vi "Configure.vi"(8 "error in (no error)":errorcluster, 11 "Cascade in":refnum<class "Cascade.lvclass">) -> (0 "error out":errorcluster, 2 "cancelled?":bool, 3 "Cascade out":refnum<class "Cascade.lvclass">)   [LabVIEW 2012, in "Cascade.lvclass"]
doc: "The configure method configures the details for the RabbitMQ connection, the observers and the mapping script.\n\nIn the derived class, make a call to the parent for setting these parameters."
uses:
  Cascade.lvclass
  timing mode.ctl
  Trigger edge.ctl
  acquire flag.ctl
  gain mode.ctl
  dependencies/ImageReg/Edge and object parameters.ctl
  dependencies/ImageReg/Registration method.ctl
  dependencies/ImageReg/BinarizationParameters.ctl
  dependencies/ImageReg/Gaussian blur parameters.ctl
  <vilib>/Utility/miscctls.llb/LVPointTypeDef.ctl
  Cascade.lvclass/Cascade.ctl
  <vilib>/Distrio/Murmex/Murmex/Murmex.lvclass
panel:
  in  "Tab Control":T1(tab)
  in  "Accumulations":u32
  in  "Number of frames":u32
  in  "Temperature":dbl=-70.0
  in  "Gain mode":T2 items=["Safe mode"=1, "Gate mode"=2, "Shutter mode"=3]
  in  "Acquire flag":T3 items=["Sync Focus mode"=1, "Sync N Frame mode"=2, "Async mode"=3, "Sequence moce"=4]
  in  "Timing mode":T4 items=["Free run"=1, "External trigger"=2, "Strobe mode  (ext trigger)"=3, "Bulb mode (ext trigger)"=4, "Variable mode (ext trigger)"=5, "Flash mdoe (ext trigger)"=6]
  in  "Trigger Edge":T5 items=["Leading edge"=1, "Falling edge"=2]
  in  "LUT":path
  in  "Background image":path
  in  "Gaussian blur parameters":T6={"large sigma"=20.0, "small sigma"=4.0, "equalize?"=FALSE}
  in  "Binarization parameters":T7={"threshold percentage"=95.0, "equalize?"=FALSE, "Method (clustering)"=0} {"Method (clustering)" items=["clustering", "entropy", "metric", "moments", "inter-class variance"]}
  in  "min physical displacement":dbl[unit]
  in  "max physical displacement":dbl[unit]
  in  "saturation limit":dbl
  in  "Registration method":T8
  in  "min y pixel displ.":dbl
  in  "max y pixel displ.":dbl
  in  "max pixel discrepancy":dbl
  in  "min x pixel displ.":dbl
  in  "max x pixel displ.":dbl
  in  "micron equivalent of pixel":dbl[unit]
  in  "brightness threshold":sgl
  in  "stage component":string
  in  "Edge and object Parameters":T9={"Canny Edge Parameters"={"Sigma"=1.0, "HThresh"=0.7, "LThres"=0.2, "WindowSize"=9}, "Smoothing parameters"={"X Size"=3, "Y Size"=3, "% Tolerance"=40}, "Dilation iteration"=1, "Object recognition parameters"={"Objects"=0, "Threshold"=128, "Reject Border"=FALSE, "Fill Holes"=FALSE, "Min Object Size"=FALSE, "Min Size"=3, "Max Object Size"=FALSE, "Max Size"=100, "Show Search Area"=FALSE, "Show Center"=TRUE, "Show Bounding Box"=TRUE}} {"Object recognition parameters"."Objects" items=["Bright Objects", "Dark Objects"]; "Object recognition parameters"."Threshold" min=1 max=999999999 step=1; "Object recognition parameters"."Max Size" min=1 max=999999999 step=1; "Object recognition parameters"."Min Size" min=1 max=999999999 step=1; "Canny Edge Parameters"."LThres" min=0 max=1 format="%.2f"; "Canny Edge Parameters"."HThresh" min=0 max=1 format="%.2f"; "Canny Edge Parameters"."Sigma" min=0 max=1 format="%.2f"}
  in  "button:call parent":bool
  in  "button:ok":bool
  in  "button:cancel":bool
  # "RabbitMQ parameters"
  # "Window position"
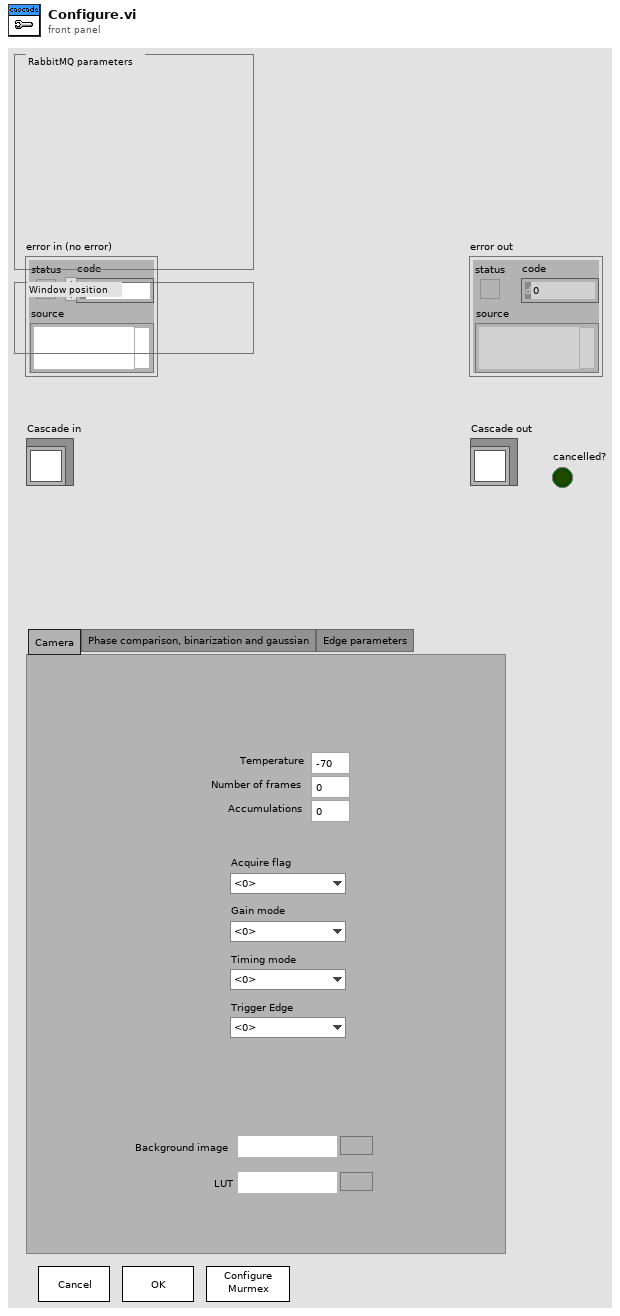
[diagram p1: front panel]
types:
  T1 = enum32{"Camera", "Phase comparison, binarization and gaussian", "Edge parameters"}
  T2 = typedef "Cascade.lvclass/gain mode.ctl" = u32
  T3 = typedef "Cascade.lvclass/acquire flag.ctl" = u32
  T4 = typedef "Cascade.lvclass/timing mode.ctl" = u32
  T5 = typedef "Cascade.lvclass/Trigger edge.ctl" = u32
  T6 = typedef "Gaussian blur parameters.ctl" = cluster{"large sigma":sgl, "small sigma":sgl, "equalize?":bool}
  T7 = typedef "BinarizationParameters.ctl" = cluster{"threshold percentage":dbl, "equalize?":bool, "Method (clustering)":i32}
  T8 = typedef "Registration method.ctl" = enum16{"Binarization", "Difference of Gaussians", "Edges Detection", "Gaussians and Binarization", "Edges and Gaussians", "Edges and Binarization", "All"}
  T9 = typedef "Edge and object parameters.ctl" = cluster{"Canny Edge Parameters":cluster{"Sigma":sgl, "HThresh":sgl, "LThres":sgl, "WindowSize":i32}, "Smoothing parameters":cluster{"X Size":i32, "Y Size":i32, "% Tolerance":i32}, "Dilation iteration":i32, "Object recognition parameters":cluster{"Objects":u16, "Threshold":i32, "Reject Border":bool, "Fill Holes":bool, "Min Object Size":bool, "Min Size":i32, "Max Object Size":bool, "Max Size":i32, "Show Search Area":bool, "Show Center":bool, "Show Bounding Box":bool}}
  T10 = typedef "LVPointTypeDef.ctl" = cluster{"Horizontal":i16, "Vertical":i16}
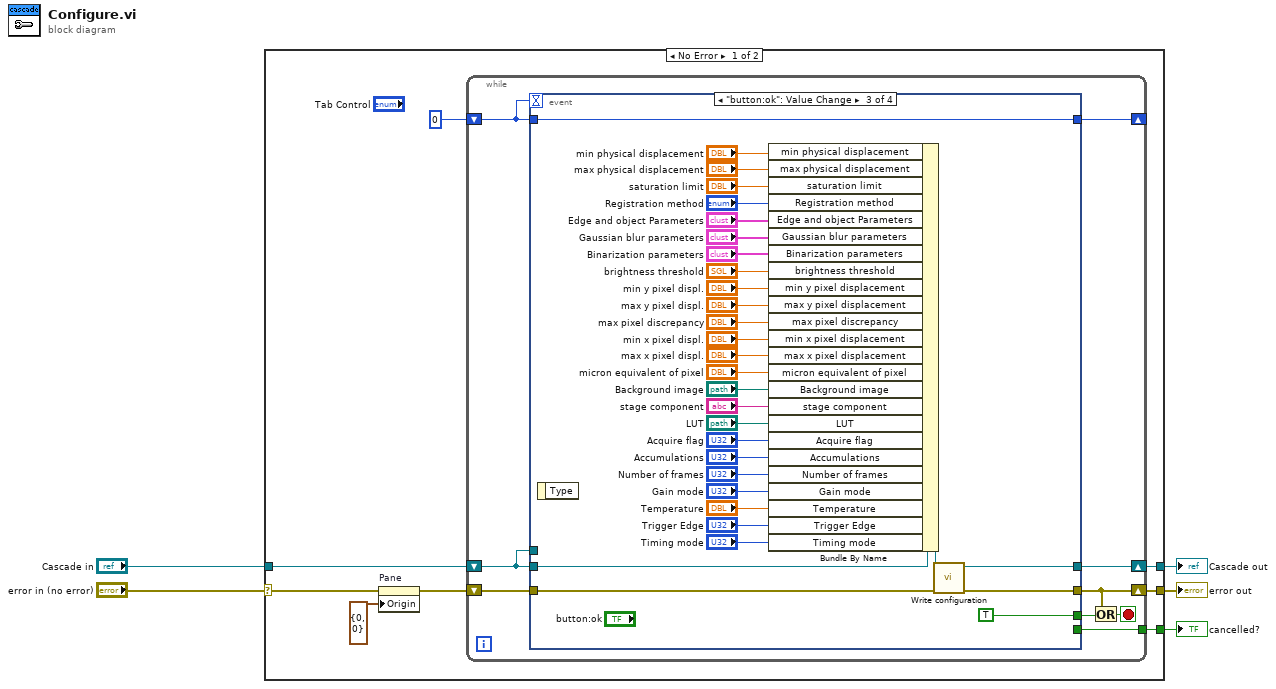
[diagram p0: block diagram]
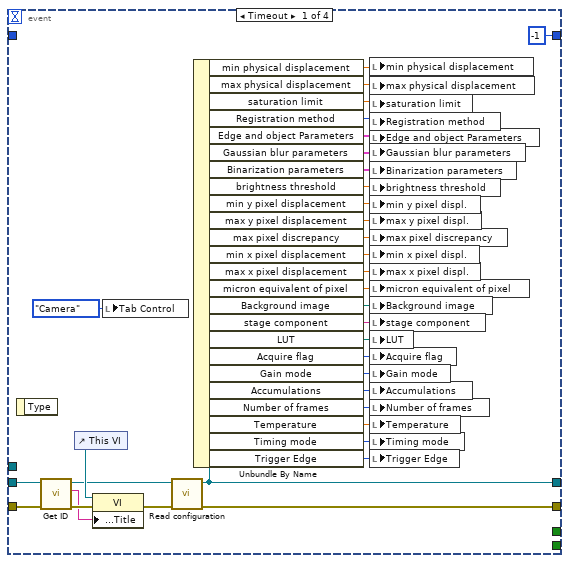
[diagram p2: hidden frame]
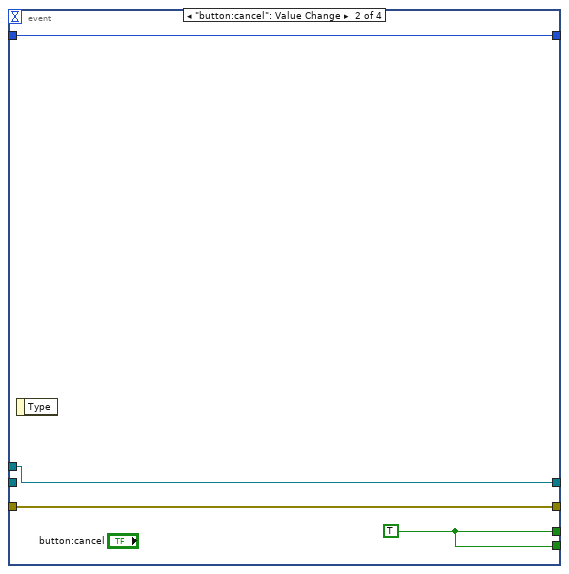
[diagram p3: hidden frame]
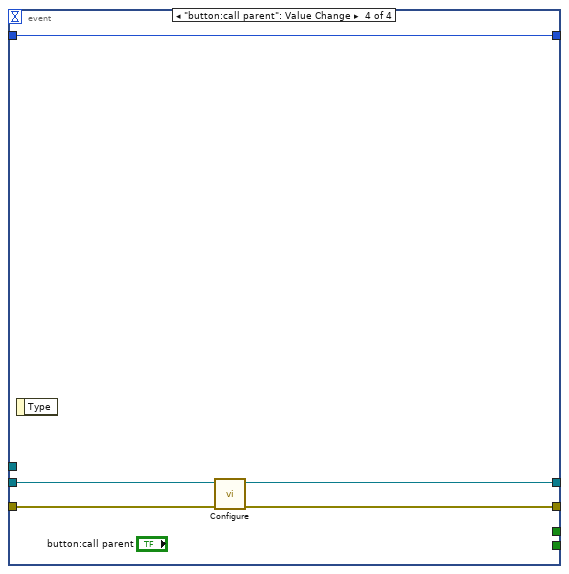
[diagram p4: hidden frame]
diagram:
  n1 = case shown="No Error" "error in (no error)" {
    selector: "error in (no error)" -> [w12 w98]
    tunnel: "Cascade in" -> [w9 w99]
    tunnel: [w10 w98] -> w3
    tunnel: [w7 w99] -> w2
    tunnel: [w6 _] -> w1
    frame No Error {
      n2 = property on="Pane" class="Pane"(error in=w12, "Origin"=T10 {"Horizontal"=0, "Vertical"=0}) -> (error out=w11:errorcluster)  [unwired: 1 in, 1 out]
      n3 = while {
        shift-right: [w17] -> w10
        shift-left: w11 -> [w22]
        shift-right: [w18] -> w7
        shift-left: w9 -> [w21]
        shift-right: [w19] -> _
        shift-left: 0 -> [w20]
        tunnel: [w14] -> w6
        stop <- w16 stop-if-true
        n4 = event shown="[2] \"button:ok\": Value Change" {
          selector: _ -> [_ _ _ _]
          dyn-events: _ -> [_ _ _ _]
          timeout: w20 -> [_ _ _ _]
          tunnel: w22 -> [w56 w60 w89 w97]
          tunnel: w21 -> [w55 _ w87 w95]
          tunnel: w21 -> [_ w61 _ _]
          tunnel: w20 -> [_ w58 w92 w93]
          tunnel: [-1 w58 w92 w93] -> w19
          tunnel: [w49 w61 w90 w94] -> w18
          tunnel: [w48 w60 w91 w96] -> w17
          tunnel: [_ w59 TRUE ("cancelled?") _] -> w15
          tunnel: [_ w59 _ _] -> w14
          event Timeout {
            n5 = event-data() -> ()  [unwired: 1 in, 1 out]
            n6 = call <vilib>:"Get ID.vi"("error in (no error)"=w56, "Murmex in"=w55) -> ("error out"=w54:errorcluster, "component id"=w50:string, "Murmex out"=w51:refnum<class "Cascade.lvclass">)  [unwired: 7 in]
            n7 = control-ref of="This VI"() -> (w53:refnum<vi>)
            n8 = property class="VI"(reference=w53, error in=w54, "Front Panel.Title"=w50) -> (error out=w52:errorcluster)  [unwired: 1 out]
            n9 = local write "Tab Control"(T1."Camera" ("Tab Control")) -> ()
            n10 = call <vilib>:"Read configuration.vi"("error in (no error)"=w52, "Murmex in"=w51) -> ("error out"=w48:errorcluster, "Murmex out"=w49:refnum<class "Cascade.lvclass">)  [unwired: 7 in, 1 out]
            n11 = Unbundle By Name(w49) -> ("min physical displacement"=w28:dbl[unit], "max physical displacement"=w29:dbl[unit], "saturation limit"=w23:dbl, "Registration method"=w24:T8, "Edge and object Parameters"=w27:T9, "Gaussian blur parameters"=w25:T6, "Binarization parameters"=w26:T7, "brightness threshold"=w31:sgl, "min y pixel displacement"=w32:dbl, "max y pixel displacement"=w33:dbl, "max pixel discrepancy"=w37:dbl, "min x pixel displacement"=w36:dbl, "max x pixel displacement"=w35:dbl, "micron equivalent of pixel"=w34:dbl[unit], "Background image"=w38:path, "stage component"=w39:string, "LUT"=w40:path, "Acquire flag"=w41:T3, "Gain mode"=w42:T2, "Accumulations"=w43:u32, "Number of frames"=w44:u32, "Temperature"=w45:dbl, "Timing mode"=w47:T4, "Trigger Edge"=w46:T5)
            n12 = local write "min physical displacement"(w28) -> ()
            n13 = local write "max physical displacement"(w29) -> ()
            n14 = local write "saturation limit"(w23) -> ()
            n15 = local write "Registration method"(w24) -> ()
            n16 = local write "Edge and object Parameters"(w27) -> ()
            n17 = local write "Gaussian blur parameters"(w25) -> ()
            n18 = local write "Binarization parameters"(w26) -> ()
            n19 = local write "brightness threshold"(w31) -> ()
            n20 = local write "min y pixel displ."(w32) -> ()
            n21 = local write "max y pixel displ."(w33) -> ()
            n22 = local write "max pixel discrepancy"(w37) -> ()
            n23 = local write "min x pixel displ."(w36) -> ()
            n24 = local write "max x pixel displ."(w35) -> ()
            n25 = local write "micron equivalent of pixel"(w34) -> ()
            n26 = local write "Background image"(w38) -> ()
            n27 = local write "stage component"(w39) -> ()
            n28 = local write "LUT"(w40) -> ()
            n29 = local write "Acquire flag"(w41) -> ()
            n30 = local write "Gain mode"(w42) -> ()
            n31 = local write "Accumulations"(w43) -> ()
            n32 = local write "Number of frames"(w44) -> ()
            n33 = local write "Temperature"(w45) -> ()
            n34 = local write "Timing mode"(w47) -> ()
            n35 = local write "Trigger Edge"(w46) -> ()
          }
          event "button:cancel": Value Change {
            w59 = TRUE ("cancelled?")
            n36 = event-data() -> ()  [unwired: 1 in, 1 out]
          }
          event "button:ok": Value Change {
            n37 = event-data() -> ()  [unwired: 1 in, 1 out]
            n38 = Bundle By Name(cluster=w87, "min physical displacement"="min physical displacement", "max physical displacement"="max physical displacement", "saturation limit"="saturation limit", "Registration method"="Registration method", "Edge and object Parameters"="Edge and object Parameters", "Gaussian blur parameters"="Gaussian blur parameters", "Binarization parameters"="Binarization parameters", "brightness threshold"="brightness threshold", "min y pixel displacement"="min y pixel displ.", "max y pixel displacement"="max y pixel displ.", "max pixel discrepancy"="max pixel discrepancy", "min x pixel displacement"="min x pixel displ.", "max x pixel displacement"="max x pixel displ.", "micron equivalent of pixel"="micron equivalent of pixel", "Background image"="Background image", "stage component"="stage component", "LUT"="LUT", "Acquire flag"="Acquire flag", "Accumulations"="Accumulations", "Number of frames"="Number of frames", "Gain mode"="Gain mode", "Temperature"="Temperature", "Trigger Edge"="Trigger Edge", "Timing mode"="Timing mode") -> (w88:refnum<class "Cascade.lvclass">)
            n39 = call <vilib>:"Write configuration.vi"("error in (no error)"=w89, "Murmex in"=w88) -> ("error out"=w91:errorcluster, "Murmex out"=w90:refnum<class "Cascade.lvclass">)  [unwired: 8 in]
          }
          event "button:call parent": Value Change {
            n40 = event-data() -> ()  [unwired: 1 in, 1 out]
            n41 = call-parent "Configure.vi"("error in (no error)"=w97, "Murmex in"=w95) -> ("error out"=w96:errorcluster, "Murmex out"=w94:refnum<class "Cascade.lvclass">)  [unwired: 7 in, 1 out]
          }
        }
        n42 = Or(x=w17, y=w15) -> (x .or. y?=w16:bool)
      }
    }
    frame Error {
    }
  }
  "error out" <- w3
  "Cascade out" <- w2
  "cancelled?" <- w1
